vi "Open Registry Key.vi"(6 "registry view":T1 items=["Default"=0, "KEY_WOW64_64KEY"=8, "KEY_WOW64_32KEY"=9], 7 "machine (local)":string, 8 "error in (no error)":errorcluster, 9 "security access mask (KEY_READ | KEY_WRITE)":T4=enum."KEY_READ | KEY_WRITE", 10 "subkey":string, 11 "root key (HKEY_LOCAL_MACHINE)":T3=enum."HKEY_LOCAL_MACHINE") -> (0 "error out":errorcluster, 3 "refnum out":T2)   [LabVIEW 2020]
doc: "Opens a reference to a key or subkey in the Windows registry."
uses:
  Registry SAM.ctl
  Registry RtKey.ctl
  Registry refnum.ctl
  Registry View.ctl
  Advapi32.dll
panel:
  in  "refnum":T2
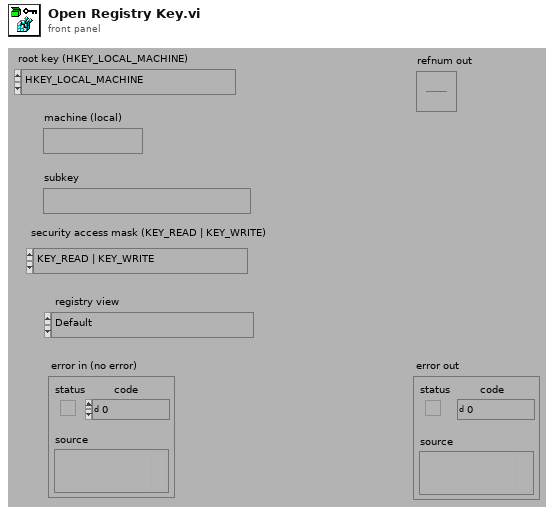
[diagram p1: front panel]
types:
  T1 = typedef "Registry View.ctl" = u16
  T2 = typedef "Registry refnum.ctl" = refnum<k1>
  T3 = typedef "Registry RtKey.ctl" = enum32{"HKEY_CLASSES_ROOT", "HKEY_CURRENT_USER", "HKEY_LOCAL_MACHINE", "HKEY_USERS", "HKEY_PERFORMANCE_DATA", "HKEY_CURRENT_CONFIG", "HKEY_DYN_DATA"}
  T4 = typedef "Registry SAM.ctl" = enum32{"KEY_QUERY_VALUE", "KEY_SET_VALUE", "KEY_CREATE_SUB_KEY", "KEY_ENUMERATE_SUB_KEYS", "KEY_NOTIFY", "KEY_CREATE_LINK", "KEY_READ", "KEY_WRITE", "KEY_ALL_ACCESS", "KEY_READ | KEY_WRITE"}
  T5 = enum16{"store handles", "dispose handles", "get handles"}
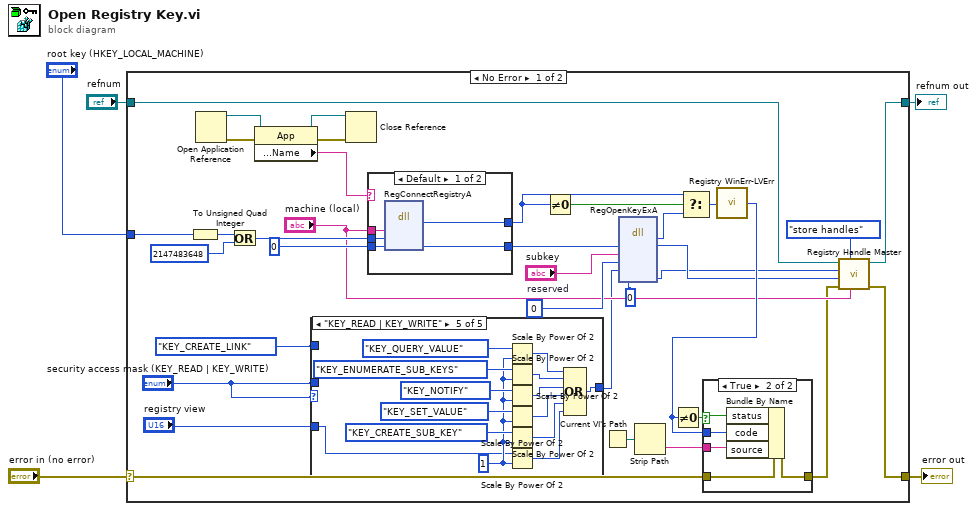
[diagram p0: block diagram]
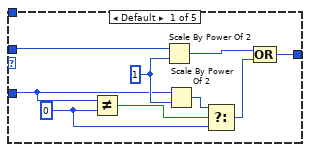
[diagram p2: hidden frame]
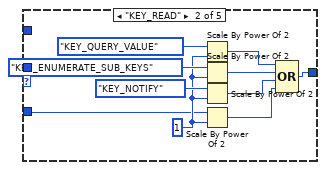
[diagram p3: hidden frame]
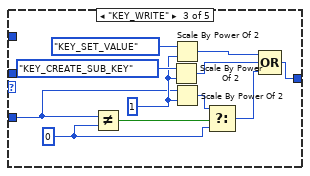
[diagram p4: hidden frame]
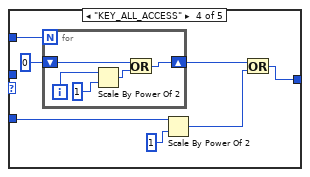
[diagram p5: hidden frame]
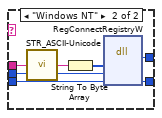
[diagram p7: hidden frame]
diagram:
  n1 = case shown="No Error" "error in (no error)" {
    selector: "error in (no error)" -> [w14 w116]
    tunnel: [w13 w116] -> w5
    tunnel: "root key (HKEY_LOCAL_MACHINE)" -> [w21 _]
    tunnel: "refnum" -> [w16 w115]
    tunnel: [w15 w115] -> w1
    frame No Error {
      w37 = u32 0  # reserved
      n2 = To Unsigned Quad Integer(1:w21) -> (0:w40:u64)
      n3 = Open Application Reference() -> (0:w25:errorcluster, 3:w26:refnum<vi>)  [unwired: 1 in, 3 out]
      n4 = Or(x=w40, y=u64 2147483648) -> (x .or. y?=w33:u64)
      n5 = property class="App"(reference=w26, error in=w25) -> (reference out=w23:refnum<vi>, error out=w24:errorcluster, "Operating System:Name"=w22:string)
      n6 = case shown="\"KEY_READ | KEY_WRITE\"" "security access mask (KEY_READ | KEY_WRITE)" {
        tunnel: [w46 w59 w66 w73 w89] -> w9
        tunnel: "security access mask (KEY_READ | KEY_WRITE)" -> [w49 _ _ _ _]
        tunnel: Registry_SAM."KEY_CREATE_LINK" ("security access mask (KEY_READ | KEY_WRITE)") -> [_ _ _ w76 _]
        tunnel: "registry view" -> [w45 w51 w64 w72 w84]
        frame Default {
          w43 = u16 0 ("y")
          w47 = u32 1
          n7 = Not Equal?(x=w45, y=w43) -> (x != y?=w44:bool)
          n8 = Scale By Power Of 2(n=w49, x=w47) -> (x*2^n=w48:u32)
          n9 = Scale By Power Of 2(n=w45, x=w47) -> (x*2^n=w42:u32)
          n10 = Select(t=w42, s=w44, f=w43) -> (s? t:f=w41:u32)
          n11 = Compound Arithmetic op=OR(w48, w41) -> (w46:u32)
        }
        frame "KEY_READ" {
          w52 = u32 1
          n12 = Scale By Power Of 2(n=Registry_SAM."KEY_QUERY_VALUE" ("security access mask (KEY_READ | KEY_WRITE)"), x=w52) -> (x*2^n=w56:u32)
          n13 = Scale By Power Of 2(n=Registry_SAM."KEY_ENUMERATE_SUB_KEYS" ("security access mask (KEY_READ | KEY_WRITE)"), x=w52) -> (x*2^n=w58:u32)
          n14 = Scale By Power Of 2(n=Registry_SAM."KEY_NOTIFY" ("security access mask (KEY_READ | KEY_WRITE)"), x=w52) -> (x*2^n=w57:u32)
          n15 = Scale By Power Of 2(n=w51, x=w52) -> (x*2^n=w50:u32)
          n16 = Compound Arithmetic op=OR(w56, w58, w57, w50) -> (w59:u32)
        }
        frame "KEY_WRITE" {
          w61 = u16 0 ("y")
          w65 = u32 1
          n17 = Not Equal?(x=w64, y=w61) -> (x != y?=w63:bool)
          n18 = Scale By Power Of 2(n=Registry_SAM."KEY_CREATE_SUB_KEY" ("security access mask (KEY_READ | KEY_WRITE)"), x=w65) -> (x*2^n=w67:u32)
          n19 = Scale By Power Of 2(n=Registry_SAM."KEY_SET_VALUE" ("security access mask (KEY_READ | KEY_WRITE)"), x=w65) -> (x*2^n=w68:u32)
          n20 = Scale By Power Of 2(n=w64, x=w65) -> (x*2^n=w62:u32)
          n21 = Select(t=w62, s=w63, f=w61) -> (s? t:f=w60:u32)
          n22 = Compound Arithmetic op=OR(w68, w67, w60) -> (w66:u32)
        }
        frame "KEY_ALL_ACCESS" {
          n23 = for {
            N: w76 -> [_]
            shift-right: [w79] -> w75
            shift-left: u32 0 -> [w80]
            i -> [w81]
            n24 = Scale By Power Of 2(n=w81, x=u32 1) -> (x*2^n=w78:u32)
            n25 = Or(x=w80, y=w78) -> (x .or. y?=w79:u32)
          }
          n26 = Scale By Power Of 2(n=w72, x=u32 1) -> (x*2^n=w71:u32)
          n27 = Or(x=w75, y=w71) -> (x .or. y?=w73:u32)
        }
        frame "KEY_READ | KEY_WRITE" {
          w85 = u32 1
          n28 = Scale By Power Of 2(n=Registry_SAM."KEY_QUERY_VALUE" ("security access mask (KEY_READ | KEY_WRITE)"), x=w85) -> (x*2^n=w94:u32)
          n29 = Scale By Power Of 2(n=Registry_SAM."KEY_ENUMERATE_SUB_KEYS" ("security access mask (KEY_READ | KEY_WRITE)"), x=w85) -> (x*2^n=w96:u32)
          n30 = Scale By Power Of 2(n=Registry_SAM."KEY_NOTIFY" ("security access mask (KEY_READ | KEY_WRITE)"), x=w85) -> (x*2^n=w95:u32)
          n31 = Scale By Power Of 2(n=Registry_SAM."KEY_SET_VALUE" ("security access mask (KEY_READ | KEY_WRITE)"), x=w85) -> (x*2^n=w88:u32)
          n32 = Scale By Power Of 2(n=Registry_SAM."KEY_CREATE_SUB_KEY" ("security access mask (KEY_READ | KEY_WRITE)"), x=w85) -> (x*2^n=w87:u32)
          n33 = Scale By Power Of 2(n=w84, x=w85) -> (x*2^n=w83:u32)
          n34 = Compound Arithmetic op=OR(w94, w96, w95, w88, w87, w83) -> (w89:u32)
        }
      }
      n35 = Close Reference(reference=w23, error in (no error)=w24) -> ()  [unwired: 1 out]
      n36 = case shown="Default" w22 {
        tunnel: "machine (local)" -> [w107 w110]
        tunnel: w33 -> [w106 w114]
        tunnel: u64 0 ("phkResult") -> [w105 w113]
        tunnel: [w104 w112] -> w31
        tunnel: [w103 w111] -> w29
        frame Default {
          n37 = dll-call lib="Advapi32.dll" fn="RegConnectRegistryA"("lpMachineName"=w107, "hKey"=w106, "phkResult"=w105) -> ("return type"=w103:i32, "phkResult"=w104:u64)  [unwired: 5 in, 2 out]
        }
        frame "Windows NT" {
          n38 = call "STR_ASCII-Unicode.vi"("ASCII string"=w110) -> ("unicode string"=w109:string)
          n39 = String To Byte Array(string=w109) -> (unsigned byte array=w108:u8[])
          n40 = dll-call lib="Advapi32.dll" fn="RegConnectRegistryW"("lpMachineName"=w108, "hKey"=w114, "phkResult"=w113) -> (w111:i32, "phkResult"=w112:u32)  [unwired: 4 in, 3 out]
        }
      }
      n41 = Not Equal To 0?(x=w29) -> (x != 0?=w30:bool)
      n42 = Current VI's Path() -> (path=w34:path)
      n43 = dll-call lib="Advapi32.dll" fn="RegOpenKeyExA"("hKey"=w31, "lpSubKey"="subkey", "uiOptions"=w37, "samDesired"=w9, "phkResult"=u64 0 ("lpcbData")) -> ("return type"=w28:i32, "hKey"=w11:u64, "phkResult"=w10:u64)  [unwired: 6 in, 2 out]
      n44 = Strip Path(path=w34) -> (name=w35:string)  [unwired: 1 out]
      n45 = Select(t=w29, s=w30, f=w28) -> (s? t:f=w27:i32)
      n46 = call "Registry WinErr-LVErr.vi"("Windows error"=w27) -> ("LabVIEW error"=w20:i32)  [unwired: 4 out]
      n47 = Not Equal To 0?(x=w20) -> (x != 0?=w19:bool)
      n48 = case shown="True" w19 {
        selector: w19 -> [_ w98]
        tunnel: w35 -> [_ w102]
        tunnel: [w97 w101] -> w12
        tunnel: w14 -> [w97 w100]
        tunnel: w20 -> [_ w99]
        frame False {
        }
        frame True {
          n49 = Bundle By Name(cluster=w100, "status"=w98, "code"=w99, "source"=w102) -> (w101:errorcluster)
        }
      }
      n50 = call "Registry Handle Master.vi"("machine"="machine (local)", "action (get handles)"=T5."store handles", "error in (no error)"=w12, "remote key handle"=w11, "key handle"=w10, "refnum"=w16) -> ("error out"=w13:errorcluster, "refnum out"=w15:T2)  [unwired: 4 out]
    }
    frame Error {
    }
  }
  "error out" <- w5
  "refnum out" <- w1
